vi "Groups - Add Group2.vi"(8 "error in (no error)":errorcluster, 9 "New Parent Group":T1, 10 "Group to Add":T1, 11 "Groups In":T1[](array[typedef])) -> (0 "error out":errorcluster, 3 "Groups Out":T1[](array[typedef]), 4 "Found and Added?":bool)   [LabVIEW 2016]
uses:
  Cluster Test/Group Data.ctl
  Cluster Test/Group Cluster.lvlib
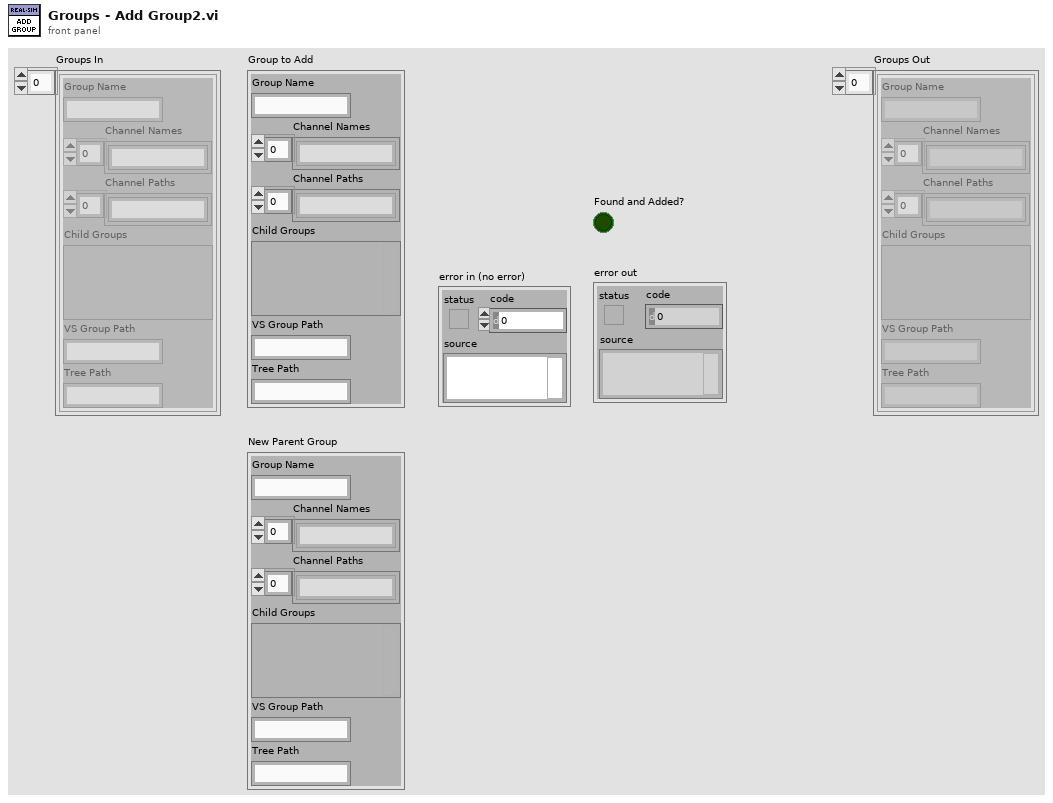
[diagram p1: front panel]
types:
  T1 = typedef "Real-Sim-Switching Shared.lvlib/Group Cluster.lvlib/Group Data.ctl" = cluster{"Group Name":string, "Channel Names":string[], "Channel Paths":string[], "Child Groups":variant, "VS Group Path":string, "Tree Path":string}
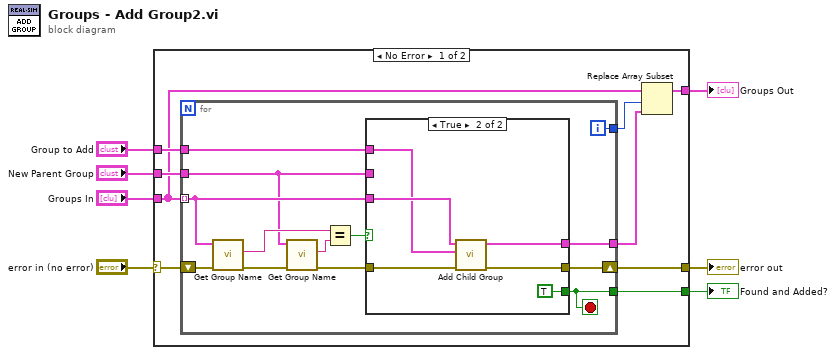
[diagram p0: block diagram]
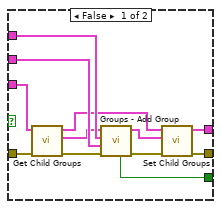
[diagram p2: hidden frame]
diagram:
  n1 = case shown="No Error" "error in (no error)" {
    selector: "error in (no error)" -> [w16 w49]
    tunnel: [w14 w49] -> w6
    tunnel: "Groups In" -> [w11 w48]
    tunnel: "New Parent Group" -> [w15 _]
    tunnel: [w8 w48] -> w1
    tunnel: [w13 _] -> w5
    tunnel: "Group to Add" -> [w12 _]
    frame No Error {
      n2 = for {
        shift-right: [w29] -> w14
        shift-left: w16 -> [w23]
        tunnel: w11 -> [w21] mode=indexing
        tunnel: [w24] -> w9
        tunnel: [w25] -> w13
        tunnel: w12 -> [w28]
        tunnel: w15 -> [w20]
        tunnel: [w26] -> w10
        i -> [w26]
        stop <- w25 stop-if-true
        n3 = call "Get Group Name.vi"("error in (no error)"=w23, "Group in"=w21) -> ("error out"=w17:errorcluster, "Group Name"=w22:string)  [unwired: 7 in, 1 out]
        n4 = call "Get Group Name.vi"("error in (no error)"=w17, "Group in"=w20) -> ("error out"=w18:errorcluster, "Group Name"=w19:string)  [unwired: 7 in, 1 out]
        n5 = Equal?(x=w22, y=w19) -> (x = y?=w27:bool)
        n6 = case shown="True" w27 {
          tunnel: w18 -> [w38 w46]
          tunnel: w21 -> [w36 w43]
          tunnel: w20 -> [w40 _]
          tunnel: [w31 w44] -> w24
          tunnel: [w34 w45] -> w29
          tunnel: [w41 TRUE ("Found and Added?")] -> w25
          tunnel: w28 -> [w39 w42]
          frame False {
            n7 = call "Get Child Groups.vi"("error in (no error)"=w38, "Group in"=w36) -> ("error out"=w37:errorcluster, "Child Groups"=w35:T1[], "Group out"=w32:T1)  [unwired: 7 in]
            n8 = call "Groups - Add Group.vi"("error in (no error)"=w37, "New Parent Group"=w40, "Group to Add"=w39, "Groups In"=w35) -> ("error out"=w33:errorcluster, "Groups Out"=w30:T1[], "Found and Added?"=w41:bool)  [unwired: 5 in]
            n9 = call "Set Child Groups.vi"("error in (no error)"=w33, "Child Groups"=w30, "Group in"=w32) -> ("error out"=w34:errorcluster, "Group out"=w31:T1)  [unwired: 7 in]
          }
          frame True {
            n10 = call "Add Child Group.vi"("error in (no error)"=w46, "Child Group"=w42, "Group in"=w43) -> ("error out"=w45:errorcluster, "Group out"=w44:T1)  [unwired: 7 in]
          }
        }
      }
      n11 = Replace Array Subset(array=w11, new element=w9, index=w10) -> (w8:T1[])
    }
    frame Error {
    }
  }
  "error out" <- w6
  "Found and Added?" <- w5
  "Groups Out" <- w1
